vi "GeneralCmd_bat.vi"(8 "COM":string="COM8", 9 "fileList_bat":path) -> (2 "file_bat":string[](array[string]))   [LabVIEW 2017]
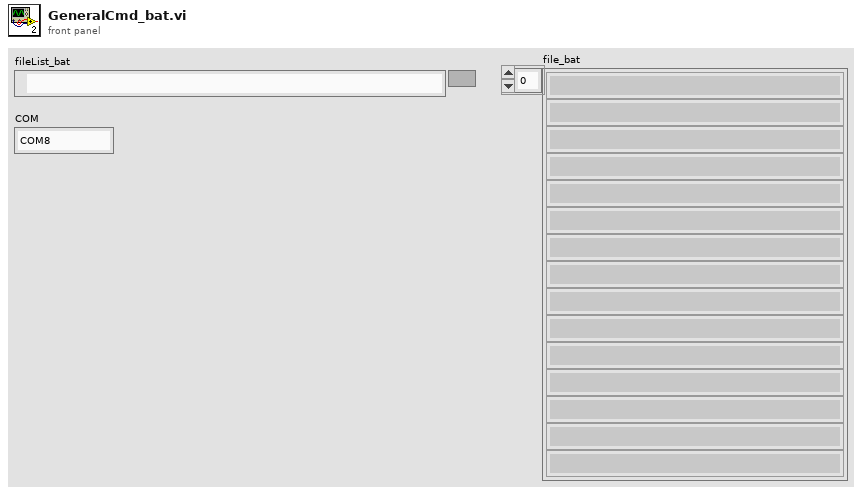
[diagram p1: front panel]
types:
  T1 = cluster{"Brush_ADC.bat":string, "Get Release Version.bat":string, "Getting Software  Version.bat":string, "Pump_ADC.bat":string, "Starting  Pump Motor.bat":string, "Starting  Test Mode.bat":string, "Starting Brush Motor 1.bat":string, "Starting Brush Motor 2.bat":string, "Starting Brush Motor 3.bat":string, "Starting LED Test.bat":string, "Stopping  Brush Motor.bat":string, "Stopping  Pump Motor.bat":string, "Stopping  Test Mode.bat":string, "1":string, "2":string, "3":string, "4":string, "5":string, "6":string, "7":string, "8":string, "9":string, "10":string}
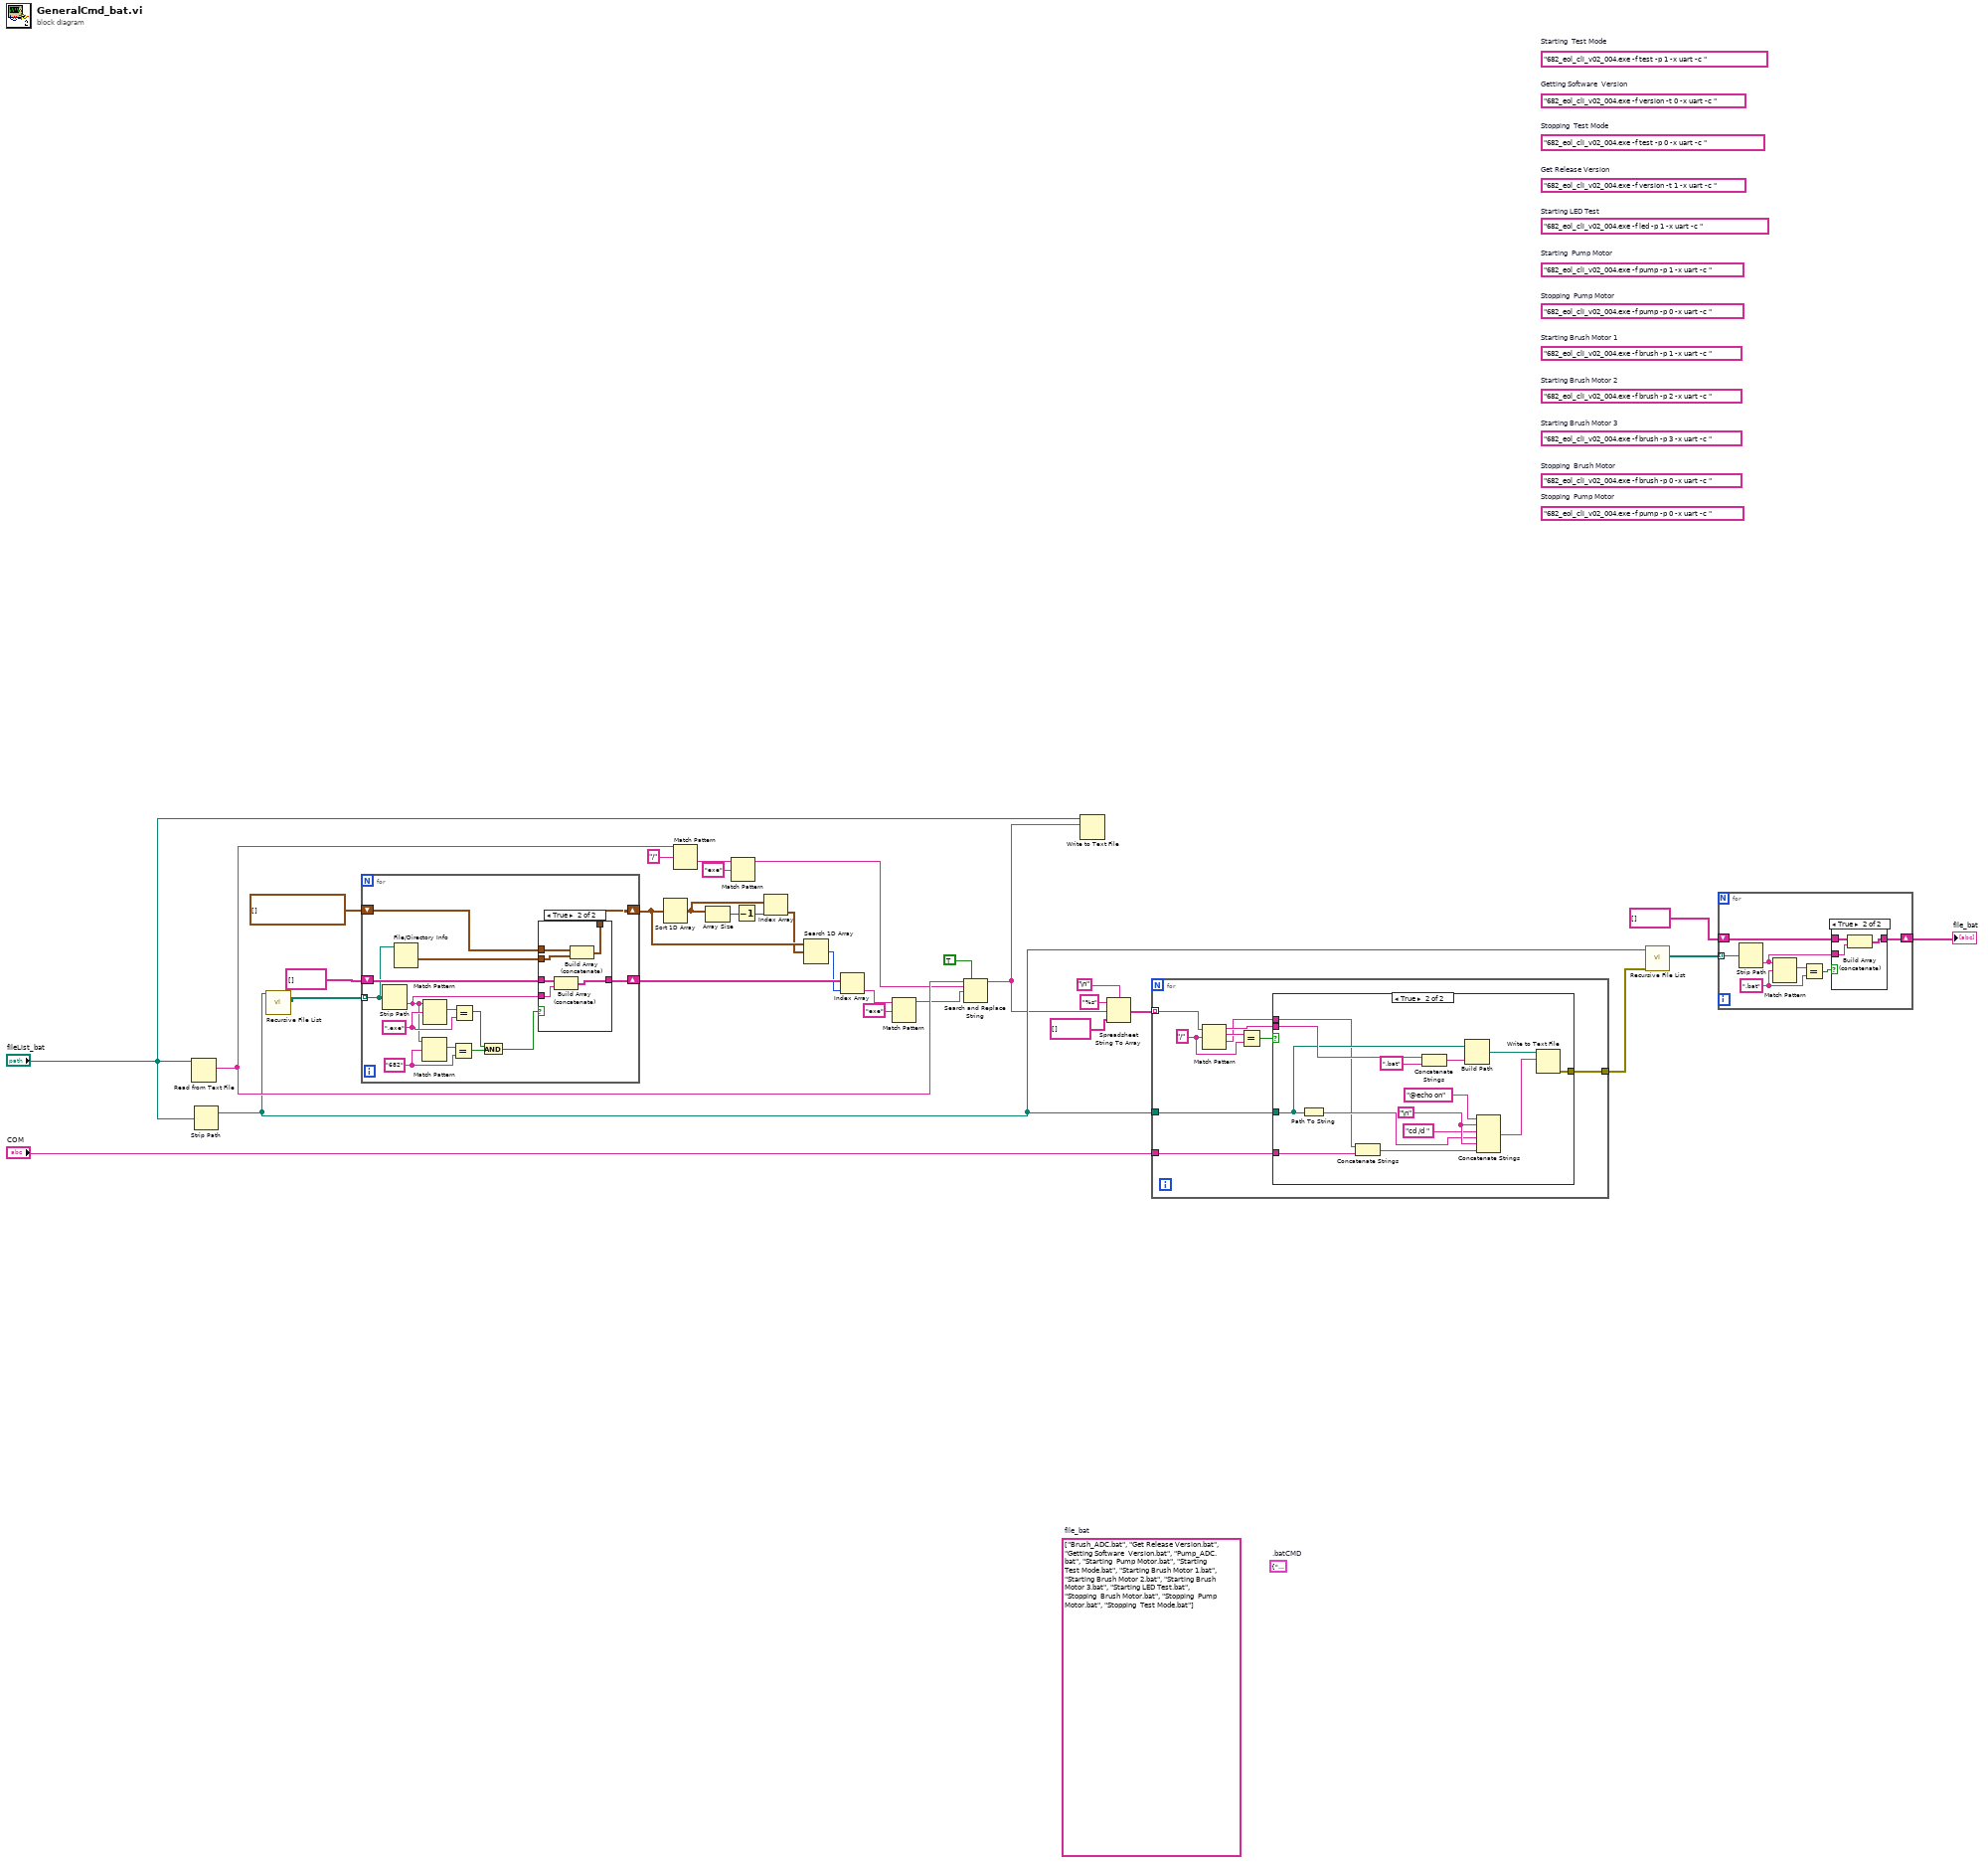
[diagram p0: block diagram]
diagram:
  (unwired) T1 {"Brush_ADC.bat"="Brush_ADC.bat", "Get Release Version.bat"="Get Release Version.bat", "Getting Software  Version.bat"="Getting Software  Version.bat", "Pump_ADC.bat"="Pump_ADC.bat", "Starting  Pump Motor.bat"="Starting  Pump Motor.bat", "Starting  Test Mode.bat"="Starting  Test Mode.bat", "Starting Brush Motor 1.bat"="Starting Brush Motor 1.bat", "Starting Brush Motor 2.bat"="Starting Brush Motor 2.bat", "Starting Brush Motor 3.bat"="Starting Brush Motor 3.bat", "Starting LED Test.bat"="Starting LED Test.bat", "Stopping  Brush Motor.bat"="Stopping  Brush Motor.bat", "Stopping  Pump Motor.bat"="Stopping  Pump Motor.bat", "Stopping  Test Mode.bat"="Stopping  Test Mode.bat", "1"="", "2"="", "3"="", "4"="", "5"="", "6"="", "7"="", "8"="", "9"="", "10"=""}  # .batCMD
  (unwired) string[] ["Brush_ADC.bat", "Get Release Version.bat", "Getting Software  Version.bat", "Pump_ADC.bat", "Starting  Pump Motor.bat", "Starting  Test Mode.bat", "Starting Brush Motor 1.bat", "Starting Brush Motor 2.bat", "Starting Brush Motor 3.bat", "Starting LED Test.bat", "Stopping  Brush Motor.bat", "Stopping  Pump Motor.bat", "Stopping  Test Mode.bat"]  # file_bat
  (unwired) "682_eol_cli_v02_004.exe -f brush -p 0 -x uart -c "  # Stopping  Brush Motor
  (unwired) "682_eol_cli_v02_004.exe -f brush -p 3 -x uart -c "  # Starting Brush Motor 3
  (unwired) "682_eol_cli_v02_004.exe -f brush -p 2 -x uart -c "  # Starting Brush Motor 2
  (unwired) "682_eol_cli_v02_004.exe -f brush -p 1 -x uart -c "  # Starting Brush Motor 1
  (unwired) "682_eol_cli_v02_004.exe -f pump -p 0 -x uart -c "  # Stopping  Pump Motor
  (unwired) "682_eol_cli_v02_004.exe -f pump -p 0 -x uart -c "  # Stopping  Pump Motor
  (unwired) "682_eol_cli_v02_004.exe -f pump -p 1 -x uart -c "  # Starting  Pump Motor
  (unwired) "682_eol_cli_v02_004.exe -f led -p 1 -x uart -c "  # Starting LED Test
  (unwired) "682_eol_cli_v02_004.exe -f version -t 1 -x uart -c "  # Get Release Version
  (unwired) "682_eol_cli_v02_004.exe -f test -p 0 -x uart -c "  # Stopping  Test Mode
  (unwired) "682_eol_cli_v02_004.exe -f test -p 1 -x uart -c "  # Starting  Test Mode
  (unwired) "682_eol_cli_v02_004.exe -f version -t 0 -x uart -c "  # Getting Software  Version
  n1 = Read from Text File(file (use dialog)="fileList_bat") -> (text=w18:string)  [unwired: 3 in, 3 out]
  n2 = Strip Path(path="fileList_bat") -> (stripped path=w15:path)  [unwired: 1 out]
  n3 = call <vilib>:"Recursive File List.vi"("Folder Path"=w15) -> ("All Files in Dir"=w14:path[])  [unwired: 6 in, 4 out]
  n4 = for {
    tunnel: w14 -> [w42] mode=indexing
    shift-right: [w43] -> w11
    shift-left: string[] [] -> [w44]
    shift-right: [w40] -> w8
    shift-left: timestamp[] [] -> [w41]
    w38 = "682" ("regular expression")
    w37 = ".exe" ("regular expression")
    n5 = Strip Path(path=w42) -> (name=w36:string)  [unwired: 1 out]
    n6 = File/Directory Info(path=w42) -> (last mod=w39:timestamp)  [unwired: 1 in, 6 out]
    n7 = Match Pattern(string=w36, regular expression=w38) -> (match substring=w32:string)  [unwired: 1 in, 3 out]
    n8 = Match Pattern(string=w36, regular expression=w37) -> (match substring=w45:string)  [unwired: 1 in, 3 out]
    n9 = Equal?(x=w32, y=w38) -> (x = y?=w35:bool)
    n10 = Equal?(x=w45, y=w37) -> (x = y?=w34:bool)
    n11 = And(x=w34, y=w35) -> (x .and. y?=w33:bool)
    n12 = case shown="True" w33 {
      tunnel: w36 -> [_ w52]
      tunnel: w44 -> [w47 w53]
      tunnel: [w47 w51] -> w43
      tunnel: w41 -> [w46 w50]
      tunnel: w39 -> [_ w49]
      tunnel: [w46 w48] -> w40
      frame False {
      }
      frame True {
        n13 = Build Array (concatenate)(w53, w52) -> (w51:string[])
        n14 = Build Array (concatenate)(w50, w49) -> (w48:timestamp[])
      }
    }
  }
  n15 = Sort 1D Array(array=w8) -> (sorted array=w10:timestamp[])
  n16 = Match Pattern(string=w18, regular expression="/") -> (after substring=w19:string)  [unwired: 1 in, 3 out]
  n17 = Array Size(array=w10) -> (size(s)=w12:i32)
  n18 = Match Pattern(string=w19, regular expression="exe") -> (before substring=w16:string)  [unwired: 1 in, 3 out]
  n19 = Decrement(x=w12) -> (x-1=w9:i32)
  n20 = Index Array(array=w10, index=w9) -> (element=w7:timestamp)
  n21 = Search 1D Array(1D array=w8, element=w7) -> (index of element=w1:i32)  [unwired: 1 in]
  n22 = Index Array(array=w11, index=w1) -> (element=w5:string)
  n23 = Match Pattern(string=w5, regular expression="exe") -> (before substring=w4:string)  [unwired: 1 in, 3 out]
  n24 = Search and Replace String(replace all?=TRUE ("replace all? (F)"), input string=w18, search string=w16, replace string=w4) -> (result string=w2:string)  [unwired: 4 in, 3 out]
  n25 = Write to Text File(file (use dialog)="fileList_bat", text=w2) -> ()  [unwired: 2 in, 3 out]
  n26 = Spreadsheet String To Array(delimiter (Tab)="\n", format string="%s", spreadsheet string=w2, array type (2D Dbl)=string[] []) -> (array=w26:string[])
  n27 = for {
    tunnel: w26 -> [w57] mode=indexing
    tunnel: w15 -> [w59]
    tunnel: [w56] -> w25
    tunnel: "COM" -> [w55]
    w61 = "/" ("regular expression")
    n28 = Match Pattern(string=w57, regular expression=w61) -> (before substring=w58:string, match substring=w62:string, after substring=w54:string)  [unwired: 1 in, 1 out]
    n29 = Equal?(x=w62, y=w61) -> (x = y?=w60:bool)
    n30 = case shown="True" w60 {
      tunnel: w59 -> [_ w69]
      tunnel: w58 -> [_ w76]
      tunnel: w54 -> [_ w63]
      tunnel: [_ w66] -> w56
      tunnel: w55 -> [_ w65]
      frame False {
      }
      frame True {
        w71 = "\n"
        n31 = Path To String(path=w69) -> (string=w67:string)
        n32 = Concatenate Strings(w63, w65) -> (w68:string)
        n33 = Concatenate Strings(w76, ".bat" ("string")) -> (w74:string)
        n34 = Build Path(base path=w69, name or relative path=w74) -> (appended path=w73:path)
        n35 = Concatenate Strings("@echo on", w71, "cd /d ", w67, w71, w68) -> (w64:string)
        n36 = Write to Text File(file (use dialog)=w73, text=w64) -> (error out=w66:errorcluster)  [unwired: 2 in, 2 out]
      }
    }
  }
  n37 = call <vilib>:"Recursive File List.vi"("error in (no error)"=w25, "Folder Path"=w15) -> ("All Files in Dir"=w22:path[])  [unwired: 5 in, 4 out]
  n38 = for {
    tunnel: w22 -> [w83] mode=indexing
    shift-right: [w77] -> w30
    shift-left: string[] [] -> [w78]
    w81 = ".bat" ("regular expression")
    n39 = Strip Path(path=w83) -> (name=w79:string)  [unwired: 1 out]
    n40 = Match Pattern(string=w79, regular expression=w81) -> (match substring=w82:string)  [unwired: 1 in, 3 out]
    n41 = Equal?(x=w82, y=w81) -> (x = y?=w80:bool)
    n42 = case shown="True" w80 {
      tunnel: w79 -> [_ w86]
      tunnel: w78 -> [w84 w87]
      tunnel: [w84 w85] -> w77
      frame False {
      }
      frame True {
        n43 = Build Array (concatenate)(w87, w86) -> (w85:string[])
      }
    }
  }
  "file_bat" <- w30
